vi "例程50-动态改变图线颜色.vi"() -> ()   [LabVIEW 2016]
uses:
  <vilib>/measure/NI_MABase.lvlib
panel:
  in  "颜色盒":u32(colorbox)=16449346
  in  "活动曲线":u32
  out "波形图表":waveform(dbl)[](graph)=[{"t0"=timestamp(212.0 s since 1904-01-01), "dt"=0.001, "Y"=array[1000 elements]}, {"t0"=timestamp(212.0 s since 1904-01-01), "dt"=0.001, "Y"=array[1000 elements]}]
  in  "停止":bool
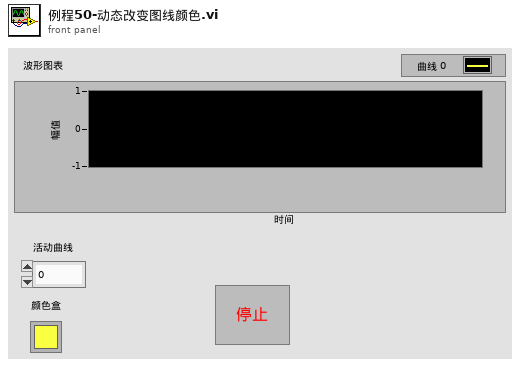
[diagram p1: front panel]
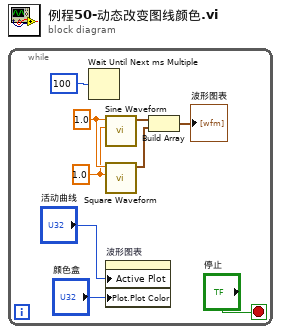
[diagram p0: block diagram]
diagram:
  n1 = while {
    stop <- "停止" stop-if-true
    w8 = 1.0 ("amplitude")
    w9 = 1.0 ("frequency")
    n2 = Wait Until Next ms Multiple(millisecond multiple=u32 100 ("毫秒倍数")) -> ()  [unwired: 1 out]
    n3 = call <vilib>:"Sine Waveform.vi"("amplitude"=w8, "frequency"=w9) -> ("signal out"=w6:waveform(dbl))  [unwired: 8 in, 1 out]
    n4 = call <vilib>:"Square Waveform.vi"("amplitude"=w8, "frequency"=w9) -> ("signal out"=w5:waveform(dbl))  [unwired: 8 in, 1 out]
    n5 = property on="波形图表" class="WFChart (严格)"("Active Plot"="活动曲线", "Plot.Plot Color"="颜色盒") -> ()  [unwired: 2 in, 2 out]
    n6 = Build Array(w6, w5) -> (→"波形图表":waveform(dbl)[])
  }
